vi "area_classes.vi"(1 "nb Class":i32=10 caption="Nb Class", 2 "CLUSTERS":i32[][](array[numeric])) -> (0 "Histogram: h(x)":i32[](array[numeric]) caption="Aires")   [LabVIEW 2018]
uses:
  <vilib>/Analysis/NI_AALBase.lvlib
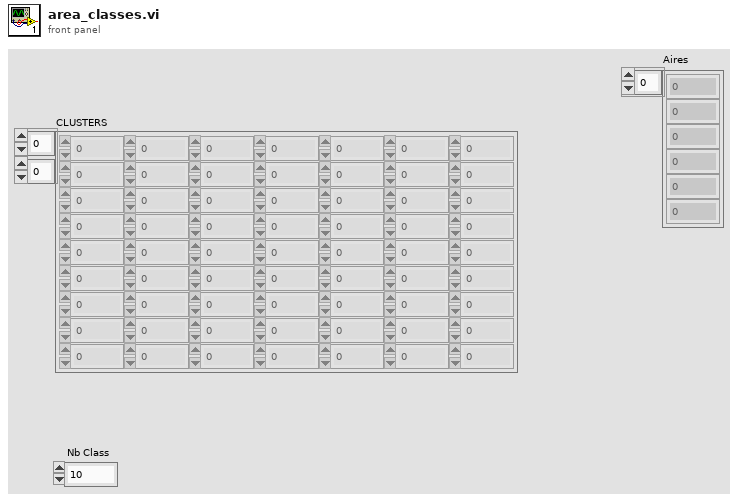
[diagram p1: front panel]
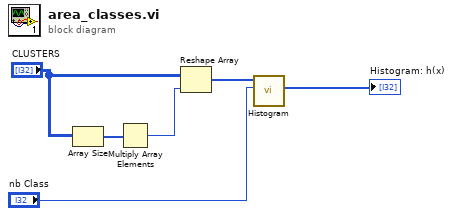
[diagram p0: block diagram]
diagram:
  n1 = Array Size(array="CLUSTERS") -> (size(s)=w6:i32[])
  n2 = Multiply Array Elements(1:w6) -> (0:w5:i32)
  n3 = Reshape Array("CLUSTERS", w5) -> (w3:i32[])
  n4 = call <vilib>:"Histogram.vi"("intervals"="nb Class", "X"=w3) -> ("Histogram: h(x)"=→"Histogram: h(x)":i32[])  [unwired: 6 in, 3 out]
